vi "Read IRQConfig.lvclass.vi"(8 "error in (no error)":errorcluster, 11 "IRQHandler in":refnum<class "IRQHandler.lvclass">) -> (0 "error out":errorcluster, 2 "IRQConfig.lvclass":refnum<class "IRQConfig.lvclass">, 3 "IRQHandler out":refnum<class "IRQHandler.lvclass">)   [LabVIEW 2013, in "ComponentData.lvlib" / "IRQHandler.lvclass"]
uses:
  <userlib>/Common/Component/common_application/RT/ComponentData/IRQHandler/IRQHandler.lvclass
  <userlib>/Common/Component/common_application/RT/ComponentData/ConfigurationHandler/IRQConfig/IRQConfig.lvclass
  <userlib>/Common/Component/common_application/RT/ComponentData/IRQHandler/IRQHandler.lvclass/IRQHandler.ctl
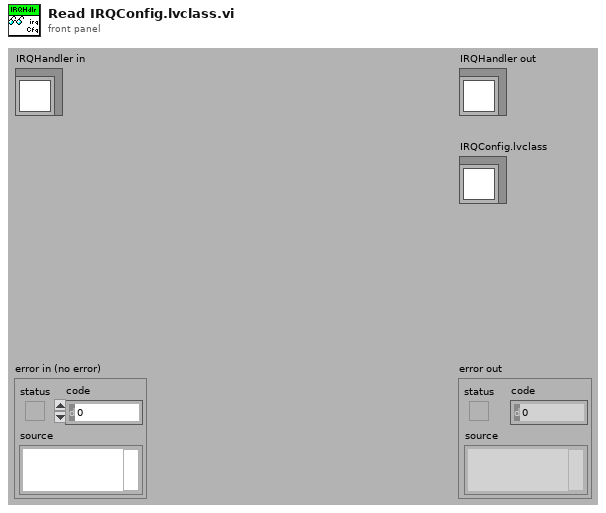
[diagram p1: front panel]
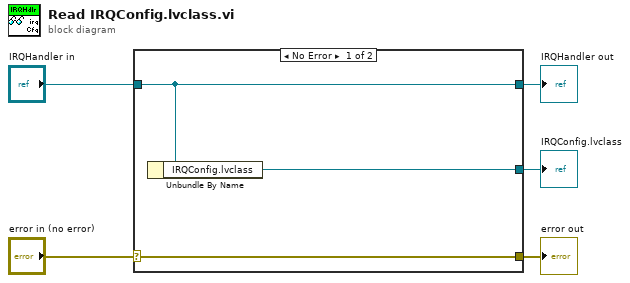
[diagram p0: block diagram]
diagram:
  n1 = case shown="No Error" "error in (no error)" {
    selector: "error in (no error)" -> [w8 w9]
    tunnel: [w8 w9] -> w4
    tunnel: [w7 w10] -> w2
    tunnel: "IRQHandler in" -> [w7 w10]
    tunnel: [w6 _] -> w1
    frame No Error {
      n2 = Unbundle By Name(w7) -> ("IRQConfig.lvclass"=w6:refnum<class "IRQConfig.lvclass">)
    }
    frame Error {
    }
  }
  "error out" <- w4
  "IRQHandler out" <- w2
  "IRQConfig.lvclass" <- w1
